vi "fg_http_configuration.vi"(7 "fg_command":T1=enum."read", 8 "error in (no error)":errorcluster, 11 "http_configuration in":T2) -> (0 "error out":errorcluster, 3 "http_configuration out":T2)   [LabVIEW 2015, in "lv-dropbox.lvlib"]
uses:
  lv-dropbox.lvlib
  _controls/http_configuration.ctl
  _controls/fg_command.ctl
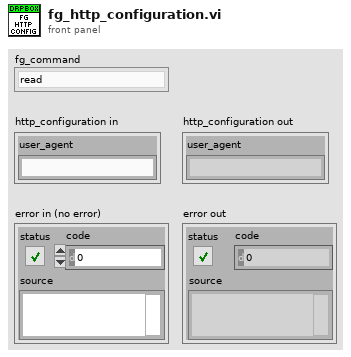
[diagram p1: front panel]
types:
  T1 = typedef "lv-dropbox.lvlib/fg_command.ctl" = enum16{"<fg_command>", "initialize", "read", "write", "shutdown"}
  T2 = typedef "lv-dropbox.lvlib/http_configuration.ctl" = cluster{"user_agent":string}
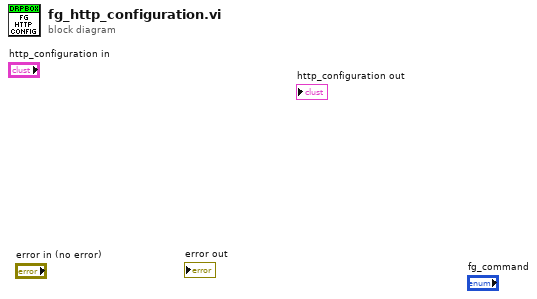
[diagram p0: block diagram]
diagram:
